vi "SpikeRemover.vi"(10 "TrigPulseWidthMin(ticks)":u64, 11 "TriggerIn":bool) -> (2 "MEasuredPulseWidth":u64, 3 "FilteredTrigger":bool)   [LabVIEW 2013]
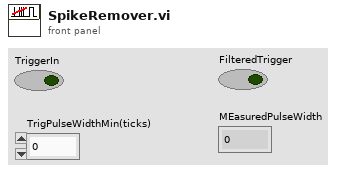
[diagram p1: front panel]
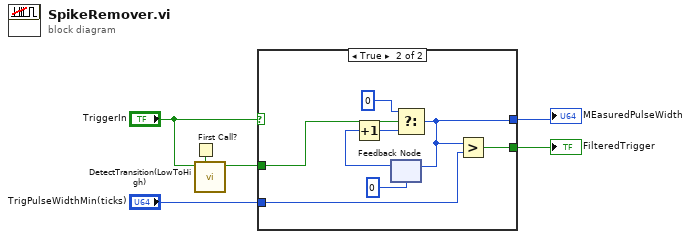
[diagram p0: block diagram]
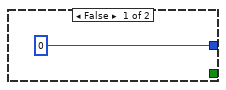
[diagram p2: hidden frame]
diagram:
  n1 = First Call?() -> (First Call?: T/F=w4:bool)
  n2 = call "DetectTransition(LowToHigh).vi"("First Call?: T/F"=w4, "InputSignal"="TriggerIn") -> ("RaisingFrontDetected"=w6:bool)  [unwired: 9 in]
  n3 = case shown="True" "TriggerIn" {
    tunnel: [_ w15] -> w2
    tunnel: "TrigPulseWidthMin(ticks)" -> [_ w9]
    tunnel: [u64 0 w10] -> w3
    tunnel: w6 -> [_ w8]
    frame False {
    }
    frame True {
      n4 = feedback #1(u64 0 ("TrigPulseWidthMin")) -> (w11:u64)
      n5 = Increment(x=w11) -> (x+1=w12:u64)
      n6 = Select(t=u64 0 ("TrigPulseWidthMin"), s=w8, f=w12) -> (s? t:f=w10:u64)
      n7 = feedback-in #1(w10) -> ()
      n8 = Greater?(x=w10, y=w9) -> (0:w15:bool)
    }
  }
  "MEasuredPulseWidth" <- w3
  "FilteredTrigger" <- w2
